vi "CollectQueueLoop.vi"(0 "reference in":refnum<class "DAQ_Base.lvclass">, 5 "error in (no error)":errorcluster) -> (14 "reference out":refnum<class "DAQ_Base.lvclass">, 19 "error out":errorcluster)   [LabVIEW 2020, in "DAQ.lvlib" / "DAQ_Base.lvclass"]
uses:
  DAQ_Base.lvclass
  E:/01_Project/CXXXX/GKN/C18726_27program_191115004/software/DAQ/DAQ_operation_type.ctl
panel:
  out "波形图":dbl[][](graph)
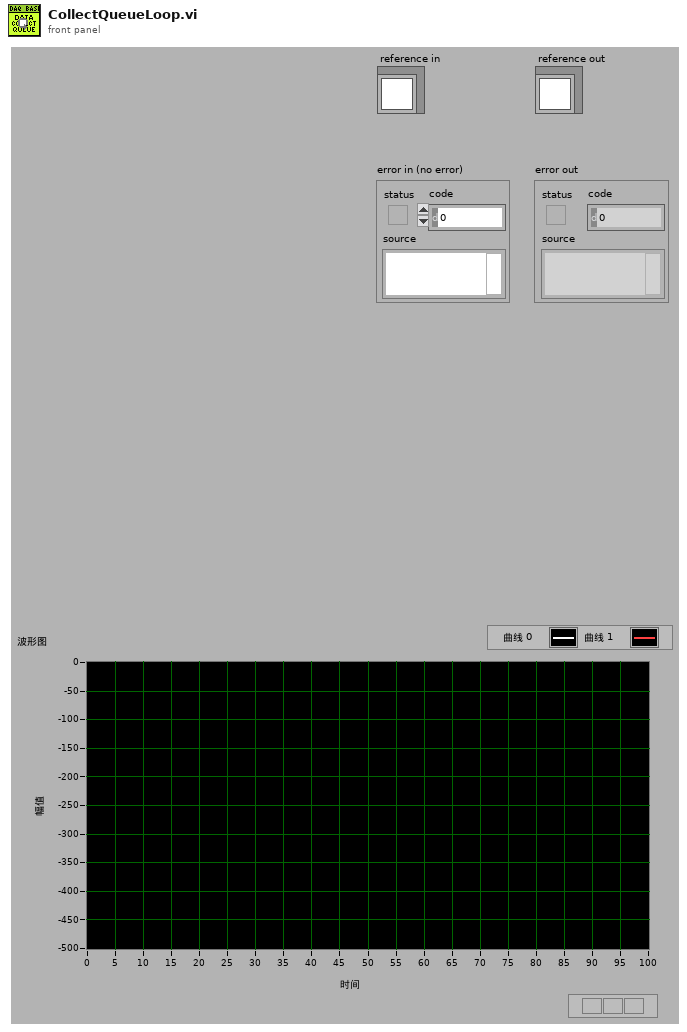
[diagram p1: front panel]
types:
  T1 = typedef "DAQ_operation_type.ctl" = enum16{"idle", "read", "write", "clear", "init", "destroy"}
  T2 = typedef "DAQ.lvlib/DAQ_Base.lvclass/ObjectAttributesRef.ctl" = refnum<data-value>
  T3 = typedef "DAQ.lvlib/DAQ_Base.lvclass/ObjectAttributes.ctl" = cluster{"MyAttribute":dbl, "RootPath":path, "DAQSettings":T4, "DaqCollector":cluster{"CollectDataQueue":refnum<queue>, "ArryDataCollectorChannel":T10[], "RealTimeValues":dbl[]}, "CollectorChannelEnable":bool[]}
  T4 = typedef "DAQ.lvlib/DAQ_Base.lvclass/DAQSettings.ctl" = cluster{"SampleSettings":T5, "AI_ChannelSettings":T6, "AO_ChannelSettings":T8, "Cnt_ChannelSettings":T9}
  T5 = typedef "DAQ.lvlib/DAQ_Base.lvclass/SampleSettings.ctl" = cluster{"samples per channel":i32, "SampleRate":dbl, "TansMaxLength":dbl, "ReadTimeOut":dbl, "时钟源":tag}
  T6 = typedef "DAQ.lvlib/DAQ_Base.lvclass/AI_ChannelSettings.ctl" = cluster{"AI_SettingsArry":cluster{"DeviceName":tag, "physical channels":tag, "AssignName":string, "输入信号类型":T7, "Max_value":dbl, "Min_value":dbl, "单位":i32, "shunt resistor location":i32, "external shunt resistor value":dbl, "标定系数":cluster{"Scale":dbl, "Offset":dbl}}[]}
  T7 = typedef "AI信号类型.ctl" = i32
  T8 = typedef "DAQ.lvlib/DAQ_Base.lvclass/AO_ChannelSettings.ctl" = cluster{"布尔":bool}
  T9 = typedef "DAQ.lvlib/DAQ_Base.lvclass/Cnt_ChannelSettings.ctl" = cluster{"Cnt_ChannelSettings":cluster{"类型":enum16{"Linear", "Rotate"}, "CounterNbr":tag, "AssignName":string, "单位":u16, "decoding type":u16, "PPR_DistancePerPulse":dbl, "Initial Position ":dbl, "z index enable":bool, "z index phase":i32, "source":tag}[]}
  T10 = typedef "DAQ.lvlib/DAQ_Base.lvclass/DataCollector.ctl" = cluster{"DataCollectArry":dbl[][], "Update":bool}
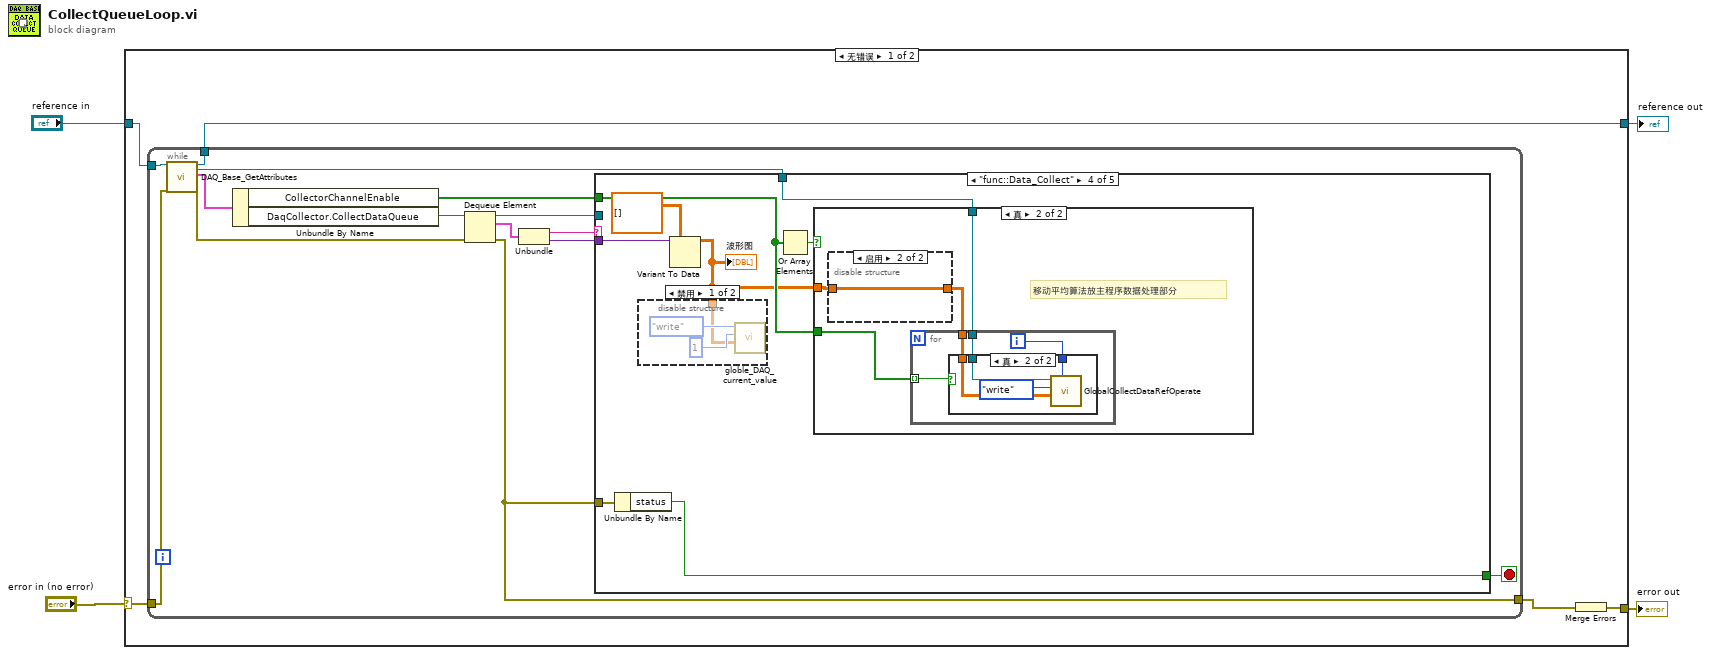
[diagram p0: block diagram]
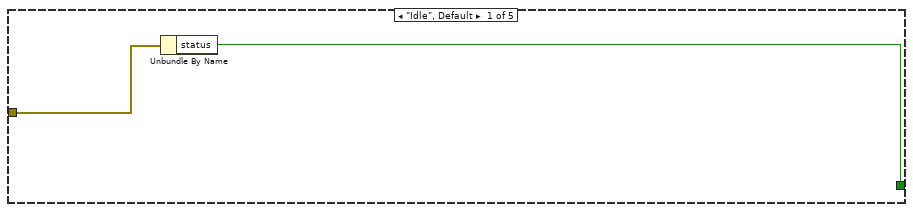
[diagram p2: hidden frame]
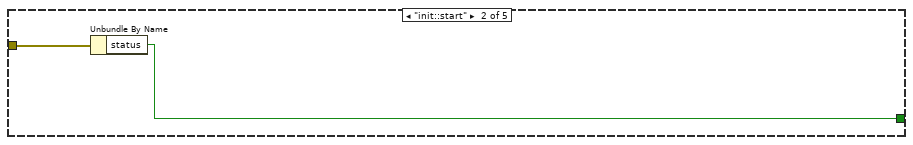
[diagram p3: hidden frame]
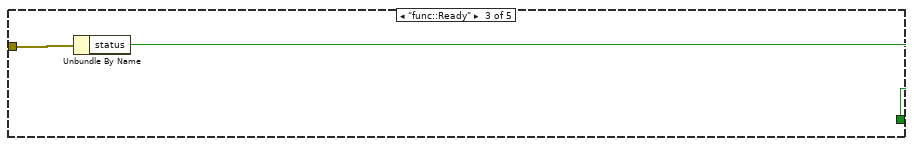
[diagram p4: hidden frame]
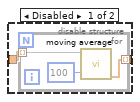
[diagram p8: hidden frame]
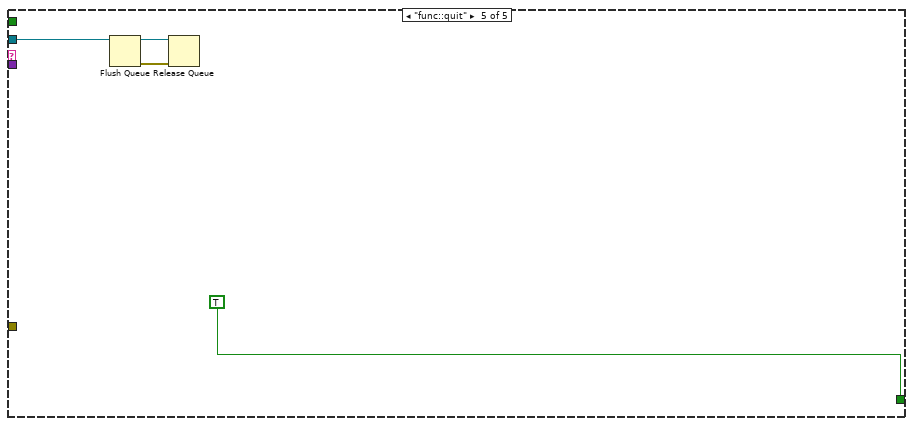
[diagram p9: hidden frame]
diagram:
  n1 = case shown="无错误" "error in (no error)" {
    selector: "error in (no error)" -> [w6 w64]
    tunnel: [w9 w64] -> w3
    tunnel: [w5 w63] -> w1
    tunnel: "reference in" -> [w7 w63]
    frame No Error {
      n2 = while {
        tunnel: [w18] -> w8
        tunnel: w7 -> [w15]
        tunnel: w6 -> [w14]
        tunnel: [w13] -> w5
        stop <- w23 stop-if-true
        n3 = call "DAQ_Base_GetAttributes.vi"("reference in"=w15, "error in (no error)"=w14) -> ("reference out"=w13:refnum<class "DAQ_Base.lvclass">, "attributes ref"=w12:T2, "attributes"=w11:T3, "error out"=w10:errorcluster)  [unwired: 14 in]
        n4 = Unbundle By Name(w11) -> ("CollectorChannelEnable"=w17:bool[], "DaqCollector.CollectDataQueue"=w16:refnum<queue>)
        n5 = Dequeue Element(queue=w16, error in (no error)=w10) -> (queue out=w19:refnum<queue>, element=w22:cluster{string, "Variant":variant}, error out=w18:errorcluster)  [unwired: 1 in, 1 out]
        n6 = Unbundle(w22) -> (w21:string, "Variant"=w20:variant)
        n7 = case shown="\"func::Data_Collect\"" w21 {
          tunnel: w20 -> [_ _ _ w37 _]
          tunnel: w19 -> [_ _ _ _ w60]
          tunnel: [w24 w26 w28 w35 TRUE] -> w23
          tunnel: w18 -> [w25 w27 w29 w36 _]
          tunnel: w17 -> [_ _ _ w32 _]
          tunnel: w12 -> [_ _ _ w30 _]
          frame "Idle", Default {
            n8 = Unbundle By Name(w25) -> ("status"=w24:bool)
          }
          frame "init::start" {
            n9 = Unbundle By Name(w27) -> ("status"=w26:bool)
          }
          frame "func::Ready" {
            n10 = Unbundle By Name(w29) -> ("status"=w28:bool)
          }
          frame "func::Data_Collect" {
            n11 = Unbundle By Name(w36) -> ("status"=w35:bool)
            n12 = Variant To Data(type=dbl[][] [] ("波形图"), Variant=w37) -> (data=w31:dbl[][])  [unwired: 1 in, 1 out]
            "波形图" <- w31
            n13 = disable-structure shown="禁用" {
              disable-tunnel: w31 -> [w38 _]
              frame Disabled {
                n14 = call "globle_DAQ_current_value.vi"("data in"=w38, "chanel_nbr"=1, "opearte"=DAQ_operation_type."write") -> ()  [unwired: 7 in, 2 out]
              }
              frame Enabled {
              }
            }
            n15 = Or Array Elements(Boolean array=w32) -> (logical OR=w33:bool)
            n16 = case shown="真" w33 {
              tunnel: w31 -> [_ w44]
              tunnel: w32 -> [_ w41]
              tunnel: w30 -> [_ w42]
              frame False {
              }
              frame True {
                # "移动平均算法放主程序数据处理部分"
                n17 = disable-structure shown="启用" {
                  disable-tunnel: w44 -> [w54 w58]
                  disable-tunnel: [w53 w58] -> w43
                  frame Disabled {
                    n18 = for {
                      tunnel: w54 -> [w57] mode=indexing
                      tunnel: [w55] -> w53 mode=indexing
                      n19 = call "moving average.vi"("Num"=100, "Filtered X"=w57) -> ("数组 2"=w55:dbl[])  [unwired: 9 in]
                    }
                  }
                  frame Enabled {
                  }
                }
                n20 = for {
                  tunnel: w43 -> [w48]
                  tunnel: w42 -> [w47]
                  tunnel: w41 -> [w45] mode=indexing
                  i -> [w46]
                  n21 = case shown="真" w45 {
                    tunnel: w48 -> [_ w52]
                    tunnel: w47 -> [_ w51]
                    tunnel: w46 -> [_ w49]
                    frame False {
                    }
                    frame True {
                      n22 = call "GlobalCollectDataRefOperate.vi"("ChannelNbr"=w49, "DatIn"=w52, "operation"=DAQ_operation_type."write" ("opearte"), "attributes ref"=w51) -> ()  [unwired: 5 in, 3 out]
                    }
                  }
                }
              }
            }
          }
          frame "func::quit" {
            n23 = Flush Queue(queue=w60) -> (queue out=w61:refnum<queue>, error out=w62:errorcluster)  [unwired: 1 in, 1 out]
            n24 = Release Queue(queue=w61, error in (no error)=w62) -> ()  [unwired: 1 in, 3 out]
          }
        }
      }
      n25 = Merge Errors(w8) -> (w9:errorcluster)
    }
    frame Error {
    }
  }
  "error out" <- w3
  "reference out" <- w1
